vi "ExperimentSettingsMenu.vi"(8 "error in (no error)":errorcluster, 11 "Small?":bool=TRUE) -> (0 "error out":errorcluster, 3 "output cluster":T1)   [LabVIEW 2013]
doc: "A menu that allows the user to select an experiment group for the current run, or create a new group and experiment."
uses:
  Controls/DisplayExperimentSetting.ctl
  <vilib>/Utility/miscctls.llb/LVPointTypeDef.ctl
  <vilib>/Utility/error.llb/DialogType.ctl
  Sub-Polymorphic/post_experiment_settings.vi
  <vilib>/addons/database/_DB Variant To Data/Database Variant To Data.xnode
panel:
  out "Experiment ID":i64
  in  "All Experiments":string[](array[string])
  out "Experiment Group":string caption="Please Enter Tags:"
  out "Experiment Name":string caption="Please Enter Tags:"
  in  "Add New Group":bool caption="OK2"
  in  "Experiment Group:":u16(ring) items=["Ablation Exp"=23, "Ablation Exp 2"=24, "Ablation Exp 3"=29, "Ablation Exp 4"=30, "Ablation Exp 5"=35, "Anna Spectrometer"=2, "BallCoatedSurfaces"=31, "Carbon Nanotubes"=33, "David Malaspina"=6, "Ejecta"=28, "Ejecta Experiments 2014"=16, "Eric Christian"=12, "Evans little thingy"=8, "Graphite Infused Peek"=32, "HyperSuda"=19, "Ice Target"=26, "June Lightflash"=1, "Keith the Drake"=7, "LDEX"=14, "Maintenance"=9, "Mehoke Foils"=15, "NDA"=3, "Negatively Charged Particles"=34, "Neutral Gas"=10, "New Group Name"=18, "November Lightflash"=5, "ODINSun"=17, "PVDF"=25, "Small Acc Dust Type Testing"=21, "Solar Cell"=13, "Stanford"=27, "STEREO"=11, "Throop Foils"=4, "Todd Bradley Florida Group"=20, "Zoltan Dust Detectors"=22]
  in  "Experiment Description:":string caption="Please Enter Experiment Description:"
  in  "New Entry":bool caption="OK2"
  in  "Cancel":bool
  in  "Experiment Name:":string caption="Please Enter Tags:"
  in  "Update Entry":bool caption="OK1"
  # "Experiment Status:"
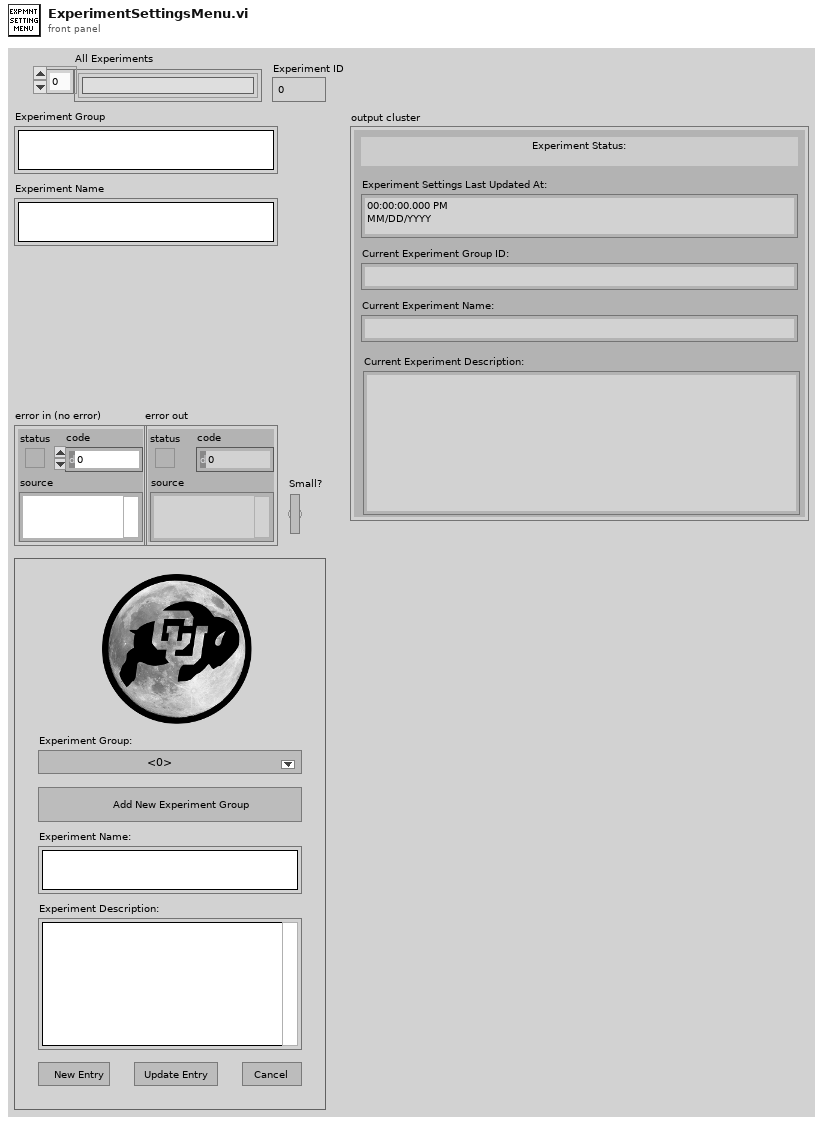
[diagram p1: front panel]
types:
  T1 = typedef "DisplayExperimentSetting.ctl" = cluster{"Current Experiment Name:":string, "Current Experiment Description:":string, "Current Experiment Group ID:":string, "Experiment Settings Last Updated At:":timestamp}
  T2 = typedef "LVPointTypeDef.ctl" = cluster{"Horizontal":i16, "Vertical":i16}
  T3 = typedef "DialogType.ctl" = u16
  T4 = typedef "LVStringsAndValuesArrayTypeDef_U16.ctl" = cluster{"String":string, "Value":u16}[]
  T5 = cluster{i64, "Integer Time":i64, "Value":u16, "Experiment Name:":string, "Experiment Description:":string}
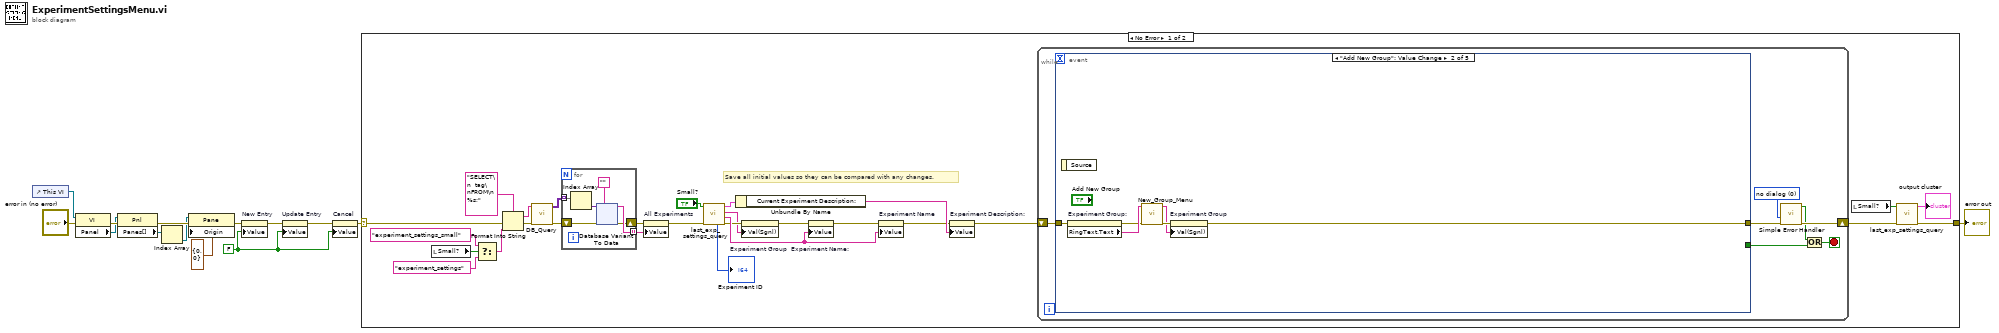
[diagram p0: block diagram]
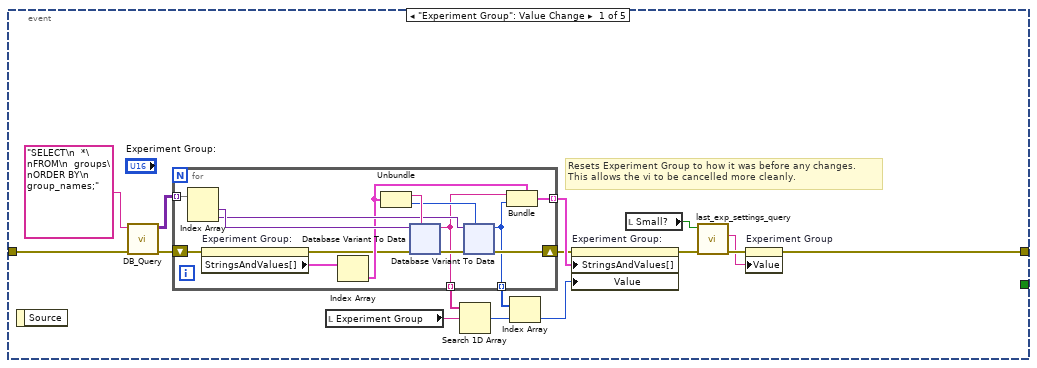
[diagram p2: hidden frame]
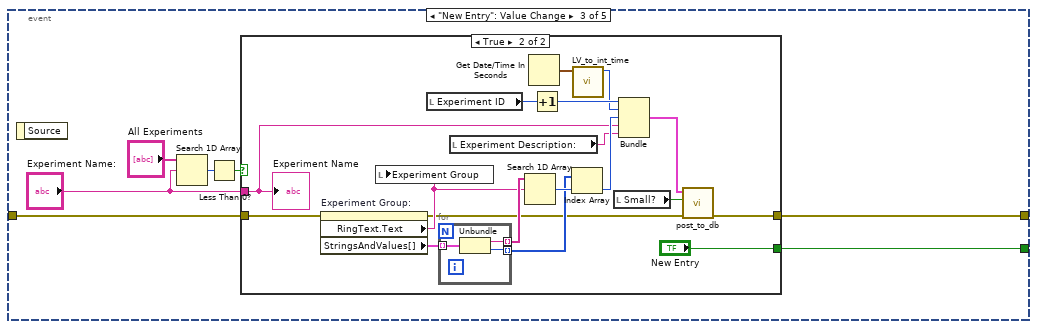
[diagram p3: hidden frame]
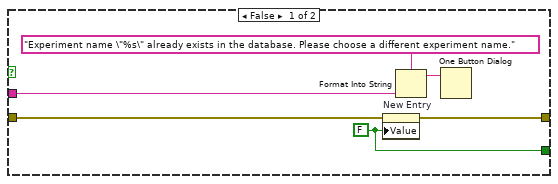
[diagram p4: hidden frame]
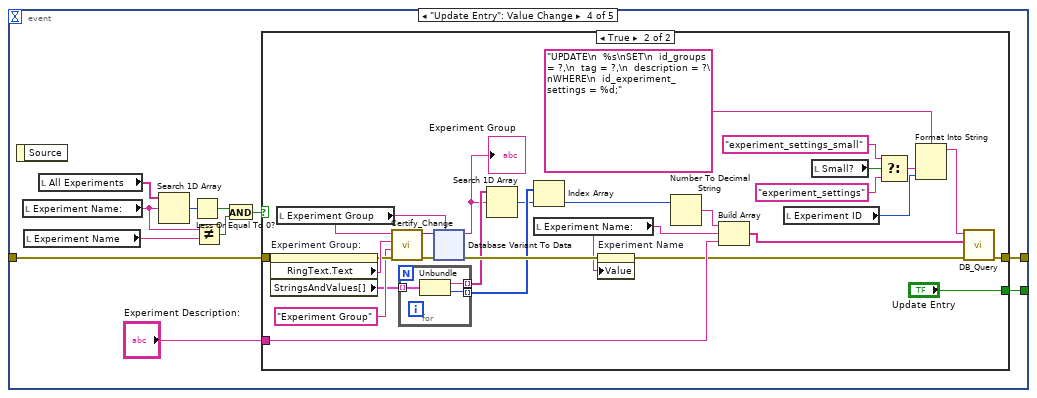
[diagram p5: hidden frame]
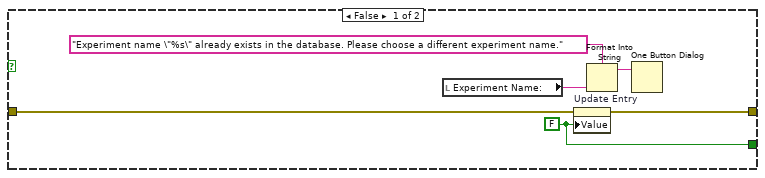
[diagram p6: hidden frame]
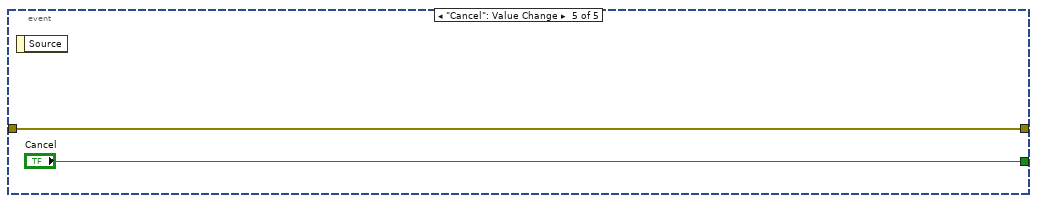
[diagram p7: hidden frame]
diagram:
  w2 = FALSE ("New Entry")
  n1 = control-ref of="This VI"() -> (w14:refnum<vi>)
  n2 = property class="VI"(reference=w14, error in="error in (no error)") -> (error out=w13:errorcluster, "Panel"=w12:refnum<vi>)  [unwired: 1 out]
  n3 = property class="Pnl"(reference=w12, error in=w13) -> (error out=w11:errorcluster, "Panes[]"=w10:refnum<vi>[])  [unwired: 1 out]
  n4 = Index Array(array=w10) -> (element=w9:refnum<vi>)  [unwired: 1 in]
  n5 = property class="Pane"(reference=w9, error in=w11, "Origin"=T2 {"Horizontal"=0, "Vertical"=0}) -> (error out=w6:errorcluster)  [unwired: 1 out]
  n6 = property on="New Entry" class="Bool (strict)"(error in=w6, "Value"=w2) -> (error out=w5:errorcluster)  [unwired: 1 in, 1 out]
  n7 = property on="Update Entry" class="Bool (strict)"(error in=w5, "Value"=w2) -> (error out=w4:errorcluster)  [unwired: 1 in, 1 out]
  n8 = property on="Cancel" class="Bool (strict)"(error in=w4, "Value"=w2) -> (error out=w3:errorcluster)  [unwired: 1 in, 1 out]
  n9 = case shown="No Error" w3 {
    selector: w3 -> [w32 w304]
    tunnel: [w22 w304] -> w1
    frame No Error {
      # "Save all initial values so they can be compared with any changes."
      n10 = local read "Small?"() -> (w35:bool)
      n11 = Select(t="experiment_settings_small", s=w35, f="experiment_settings") -> (s? t:f=w36:string)
      n12 = Format Into String(format string="SELECT\n  tag\nFROM\n  %s;" ("Parameterized Query"), error in=w32, w36) -> (resulting string=w38:string, error out=w39:errorcluster)  [unwired: 1 in]
      n13 = call "DB_Query.vi"("error in (no error)"=w39, "Parameterized Query"=w38) -> ("error out"=w31:errorcluster, "Results"=w30:variant[][])  [unwired: 7 in, 1 out]
      n14 = for {
        shift-right: [w43] -> w28
        shift-left: w31 -> [w47]
        tunnel: w30 -> [w45] mode=indexing
        tunnel: [w44] -> w27 mode=indexing
        n15 = Index Array(array=w45) -> (element=w48:variant)  [unwired: 1 in]
        n16 = xnode "Database Variant To Data"("database variant"=w48, "error in (no error)"=w47, "type"="") -> ("data"=w44:string, "error out"=w43:errorcluster)
      }
      n17 = property on="All Experiments" class="Arr (strict)"(error in=w28, "Value"=w27) -> (error out=w29:errorcluster)  [unwired: 1 in, 1 out]
      n18 = call "last_exp_settings_query.vi"("error in (no error)"=w29, "Small?"="Small?") -> ("error out"=w25:errorcluster, "Experiment Name"=w40:string, "Group Name"=w15:string, "Experiment Settings"=w16:T1, "Experiment ID"=→"Experiment ID":i64)  [unwired: 4 in, 1 out]
      n19 = Unbundle By Name(w16) -> ("Current Experiment Description:"=w24:string)
      n20 = property on="Experiment Group" class="Str"(error in=w25, "Val(Sgnl)"=w15) -> (error out=w19:errorcluster)  [unwired: 1 in, 1 out]
      n21 = property on="Experiment Name:" class="Str"(error in=w19, "Value"=w40) -> (error out=w42:errorcluster)  [unwired: 1 in, 1 out]
      n22 = property on="Experiment Name" class="Str"(error in=w42, "Value"=w40) -> (error out=w18:errorcluster)  [unwired: 1 in, 1 out]
      n23 = property on="Experiment Description:" class="Str"(error in=w18, "Value"=w24) -> (error out=w17:errorcluster)  [unwired: 1 in, 1 out]
      n24 = while {
        shift-right: [w84] -> w23
        shift-left: w17 -> [w87]
        stop <- w83 stop-if-true
        w81 = T3 0 items=["no dialog", "OK message", "continue or stop message", "OK message + warnings", "continue/stop + warnings"] ("type of dialog (OK msg:1)")
        n25 = event shown="[1] \"Add New Group\": Value Change" {
          selector: _ -> [_ _ _ _ _]
          dyn-events: _ -> [_ _ _ _ _]
          timeout: _ -> [_ _ _ _ _]
          tunnel: w87 -> [w90 w186 w188 w229 w302]
          tunnel: [w92 w182 w190 w232 w302] -> w86
          tunnel: [_ _ w189 w231 "Cancel"] -> w85
          event "Experiment Group": Value Change {
            # "Resets Experiment Group to how it was before any changes.\nThis allows the vi to be cancelled more cleanly."
            n26 = event-data() -> ()  [unwired: 1 in, 1 out]
            n27 = call "DB_Query.vi"("error in (no error)"=w90, "Parameterized Query"="SELECT\n  *\nFROM\n  groups\nORDER BY\n  group_names;") -> ("error out"=w96:errorcluster, "Results"=w97:variant[][])  [unwired: 7 in, 1 out]
            n28 = for {
              shift-right: [w108] -> w98
              shift-left: w96 -> [w105]
              tunnel: w97 -> [w117] mode=indexing
              tunnel: [w109] -> w99 mode=indexing
              tunnel: [w107] -> w100 mode=indexing
              tunnel: [w106] -> w102 mode=indexing
              n29 = Index Array(array=w117) -> (element #1=w114:variant, element #2=w112:variant)  [unwired: 2 in]
              n30 = property on="Experiment Group:" class="Ring (strict)"(error in=w105) -> (error out=w104:errorcluster, "StringsAndValues[]"=w116:T4)  [unwired: 1 in, 1 out]
              n31 = Index Array(array=w116) -> (element=w111:cluster{"String":string, "Value":u16})  [unwired: 1 in]
              n32 = Unbundle(w111) -> ("String"=w115:string, "Value"=w113:u16)
              n33 = xnode "Database Variant To Data"("database variant"=w114, "error in (no error)"=w104, "type"=w115) -> ("data"=w107:string, "error out"=w110:errorcluster)
              n34 = xnode "Database Variant To Data"("database variant"=w112, "error in (no error)"=w110, "type"=w113) -> ("data"=w106:u16, "error out"=w108:errorcluster)
              n35 = Bundle(cluster=w111, "String"=w107, "Value"=w106) -> (w109:cluster{"String":string, "Value":u16})
            }
            n36 = local read "Experiment Group"() -> (w89:string)
            n37 = Search 1D Array(1D array=w100, element=w89) -> (index of element=w101:i32)  [unwired: 1 in]
            n38 = Index Array(array=w102, index=w101) -> (element=w103:u16)
            n39 = property on="Experiment Group:" class="Ring (strict)"(error in=w98, "StringsAndValues[]"=w99, "Value"=w103) -> (error out=w93:errorcluster)  [unwired: 1 in, 1 out]
            n40 = local read "Small?"() -> (w91:bool)
            n41 = call "last_exp_settings_query.vi"("error in (no error)"=w93, "Small?"=w91) -> ("error out"=w94:errorcluster, "Group Name"=w88:string)  [unwired: 4 in, 4 out]
            n42 = property on="Experiment Group" class="Str"(error in=w94, "Value"=w88) -> (error out=w92:errorcluster)  [unwired: 1 in, 1 out]
          }
          event "Add New Group": Value Change {
            n43 = event-data() -> ()  [unwired: 1 in, 1 out]
            n44 = property on="Experiment Group:" class="Ring (strict)"(error in=w186) -> (error out=w185:errorcluster, "RingText.Text"=w187:string)  [unwired: 1 in, 1 out]
            n45 = call "New_Group_Menu.vi"("error in (no error)"=w185, "Default Name"=w187) -> ("error out"=w184:errorcluster, "Group Name"=w183:string)  [unwired: 8 in]
            n46 = property on="Experiment Group" class="Str"(error in=w184, "Val(Sgnl)"=w183) -> (error out=w182:errorcluster)  [unwired: 1 in, 1 out]
          }
          event "New Entry": Value Change {
            n47 = event-data() -> ()  [unwired: 1 in, 1 out]
            n48 = Search 1D Array(1D array="All Experiments", element="Experiment Name:") -> (index of element=w193:i32)  [unwired: 1 in]
            n49 = Less Than 0?(x=w193) -> (x < 0?=w194:bool)
            n50 = case shown="True" w194 {
              tunnel: [w197 w207] -> w190
              tunnel: [w196 "New Entry"] -> w189
              tunnel: "Experiment Name:" -> [w198 w210]
              tunnel: w188 -> [w195 w204]
              frame False {
                w196 = FALSE ("New Entry")
                n51 = property on="New Entry" class="Bool (strict)"(error in=w195, "Value"=w196) -> (error out=w197:errorcluster)  [unwired: 1 in, 1 out]
                n52 = Format Into String(format string="Experiment name \"%s\" already exists in the database. Please choose a different experiment name.", w198) -> (resulting string=w199:string)  [unwired: 2 in, 1 out]
                n53 = One Button Dialog(message=w199) -> ()  [unwired: 1 in, 1 out]
              }
              frame True {
                n54 = property on="Experiment Group:" class="Ring (strict)"(error in=w204) -> (error out=w206:errorcluster, "RingText.Text"=w208:string, "StringsAndValues[]"=w209:T4)  [unwired: 1 in, 1 out]
                n55 = local write "Experiment Group"(w208) -> ()
                n56 = local read "Experiment ID"() -> (w203:i64)
                n57 = for {
                  tunnel: w209 -> [w221] mode=indexing
                  tunnel: [w220] -> w213 mode=indexing
                  tunnel: [w219] -> w212 mode=indexing
                  n58 = Unbundle(w221) -> ("String"=w220:string, "Value"=w219:u16)
                }
                n59 = local read "Experiment Description:"() -> (w201:string)
                n60 = Search 1D Array(1D array=w213, element=w208) -> (index of element=w214:i32)  [unwired: 1 in]
                n61 = Get Date/Time In Seconds() -> (seconds since 1Jan1904=w217:timestamp)
                n62 = Increment(x=w203) -> (x+1=w216:i64)
                n63 = Index Array(array=w212, index=w214) -> (element=w211:u16)
                n64 = call "LV_to_int_time.vi"("Time Stamp"=w217) -> ("Integer Time"=w215:i64)  [unwired: 8 in, 1 out]
                n65 = local read "Small?"() -> (w205:bool)
                n66 = Bundle(w216, "Integer Time"=w215, "Value"=w211, "Experiment Name:"=w210, "Experiment Description:"=w201) -> (w202:T5)  [unwired: 1 in]
                n67 = call-poly "post_to_db.vi"("error in (no error)"=w206, "Small?"=w205, "Cluster"=w202) -> ("error out"=w207:errorcluster)  [unwired: 8 in]
                "Experiment Name" <- w210
              }
            }
          }
          event "Update Entry": Value Change {
            n68 = event-data() -> ()  [unwired: 1 in, 1 out]
            n69 = local read "Experiment Name:"() -> (w223:string)
            n70 = local read "Experiment Name"() -> (w222:string)
            n71 = local read "All Experiments"() -> (w225:string[])
            n72 = Search 1D Array(1D array=w225, element=w223) -> (index of element=w226:i32)  [unwired: 1 in]
            n73 = Less Or Equal To 0?(x=w226) -> (x <= 0?=w227:bool)
            n74 = Not Equal?(x=w223, y=w222) -> (x != y?=w224:bool)
            n75 = And(x=w227, y=w224) -> (x .and. y?=w228:bool)
            n76 = case shown="True" w228 {
              tunnel: [w236 w265] -> w232
              tunnel: [w235 "Update Entry"] -> w231
              tunnel: "Experiment Description:" -> [_ w264]
              tunnel: w229 -> [w234 w249]
              frame False {
                w235 = FALSE ("New Entry")
                n77 = local read "Experiment Name:"() -> (w233:string)
                n78 = property on="Update Entry" class="Bool (strict)"(error in=w234, "Value"=w235) -> (error out=w236:errorcluster)  [unwired: 1 in, 1 out]
                n79 = Format Into String(format string="Experiment name \"%s\" already exists in the database. Please choose a different experiment name.", w233) -> (resulting string=w237:string)  [unwired: 2 in, 1 out]
                n80 = One Button Dialog(message=w237) -> ()  [unwired: 1 in, 1 out]
              }
              frame True {
                n81 = property on="Experiment Group:" class="Ring (strict)"(error in=w249) -> (error out=w251:errorcluster, "RingText.Text"=w252:string, "StringsAndValues[]"=w245:T4)  [unwired: 1 in, 1 out]
                n82 = local read "Experiment Group"() -> (w255:string)
                n83 = call "Certify_Change.vi"("error in (no error)"=w251, "Variable Name"="Experiment Group", "New Value"=w252, "Default Value"=w255) -> ("error out"=w254:errorcluster, "Value Out"=w253:variant)  [unwired: 6 in]
                n84 = for {
                  tunnel: w245 -> [w269] mode=indexing
                  tunnel: [w268] -> w242 mode=indexing
                  tunnel: [w267] -> w244 mode=indexing
                  n85 = Unbundle(w269) -> ("String"=w268:string, "Value"=w267:u16)
                }
                n86 = xnode "Database Variant To Data"("database variant"=w253, "error in (no error)"=w254, "type"=w255) -> ("data"=w241:string, "error out"=w248:errorcluster)
                "Experiment Group" <- w241
                n87 = Search 1D Array(1D array=w242, element=w241) -> (index of element=w243:i32)  [unwired: 1 in]
                n88 = Index Array(array=w244, index=w243) -> (element=w240:u16)
                n89 = local read "Experiment Name:"() -> (w247:string)
                n90 = property on="Experiment Name" class="Str"(error in=w248, "Value"=w247) -> (error out=w262:errorcluster)  [unwired: 1 in, 1 out]
                n91 = Number To Decimal String(number=w240) -> (decimal integer string=w246:string)  [unwired: 1 in]
                n92 = Build Array(w246, w247, w264) -> (w263:string[])
                n93 = local read "Experiment ID"() -> (w239:i64)
                n94 = local read "Small?"() -> (w259:bool)
                n95 = Select(t="experiment_settings_small", s=w259, f="experiment_settings") -> (s? t:f=w260:string)
                n96 = Format Into String(format string="UPDATE\n  %s\nSET\n  id_groups = ?,\n  tag = ?,\n  description = ?\nWHERE\n  id_experiment_settings = %d;" ("Parameterized Query"), w260, w239) -> (resulting string=w256:string)  [unwired: 2 in, 1 out]
                n97 = call "DB_Query.vi"("error in (no error)"=w262, "Parameters"=w263, "Parameterized Query"=w256) -> ("error out"=w265:errorcluster)  [unwired: 6 in, 2 out]
              }
            }
          }
          event "Cancel": Value Change {
            n98 = event-data() -> ()  [unwired: 1 in, 1 out]
          }
        }
        n99 = call <vilib>:"Simple Error Handler.vi"("type of dialog (OK msg:1)"=w81, "error in (no error)"=w86) -> ("error?"=w82:bool, "error out"=w84:errorcluster)  [unwired: 3 in, 3 out]
        n100 = Or(x=w82, y=w85) -> (x .or. y?=w83:bool)
      }
      n101 = local read "Small?"() -> (w20:bool)
      n102 = call "last_exp_settings_query.vi"("error in (no error)"=w23, "Small?"=w20) -> ("error out"=w22:errorcluster, "Experiment Settings"=→"output cluster":T1)  [unwired: 4 in, 4 out]
    }
    frame Error {
    }
  }
  "error out" <- w1
